vi "FRF_Query.vi"(0 "System no.":i32=1 min=1 max=4 step=1, 2 "Axes to query":string[](array[string]), 3 "All axes?":bool, 4 "Axis identifier?":bool=TRUE, 5 "error in":errorcluster) -> (14 "Referenced?":bool[](array[boolean]), 19 "error out":errorcluster)   [LabVIEW 2020]
doc: "GCS 3.0\n=====\n\nFRF? (Get Referencing Result) \n\nDescription \nQueries whether the axes are referenced.\n\nFormat\nFRF?[ <AxisID>]\n\nArguments\nFRF without arguments starts a reference move for all axes of the controller. The axes start \nsimultaneously.\n<AxisID>\nAn axis of the controller\nThe response to USG? CMD FRF? indicates in the #Related Units block for which axes the \ncommand can be used.\nPossible values: Alias of the axis (p. 94) \n\nResponse\n{<AxisID>\"=\"<Ref_State> LF}\n<Ref_State>\nValue that indicates whether the axis is referenced.\nPossible values:\n0 = Axis is not referenced\n1 = Axis is referenced\n\nExample\n>>frf?\n<<AXIS_1=1\n<<AXIS_2=0\n\nNotes\nWhether the axis is referenced is also displayed in the status register of the axis, which can be \nqueried with the STV? command. \n\nUser command level\nUSR\n\n\nGCS 2.0\n=====\n\nIndicates whether queried axes have been referenced (using REF, FNL, FPL, FRF, MPL, MNL, or - if reference mode is OFF - using POS) successfully or not.\n\nC-413, C-843, C-843.PM, C-866, C-867, C-877, C-880, C-884, C-885, C-886, C-891, E-754, E-861, E-871, E-873, E-874, Hydra, Pollux, Mercury_GCS: If All axes? = TRUE, then Axis identifier? can be FALSE\n\nC-880K005: VI only supported when called through PI_Multix.vi\n\nE-712: If All axes? = TRUE, then Axis identifier? can be FALSE. \n\nE-755: If All axes? = TRUE, then Axis identifier? can be FALSE. Command not available for E-755.101\n\nC-887, F-206, M-8X0: If All axes? = TRUE, then Axis identifier? can be FALSE. Only for GCS syntax version = GCS 2.0 or higher (check with CSV?.vi. If CSV?.vi is not supported, syntax version is GCS 1.0)."
panel:
  # "FRF? (Get Referencing Result)\n\nQueries whether the axes are referenced."
  # "Query"
  # "If all axes: use"
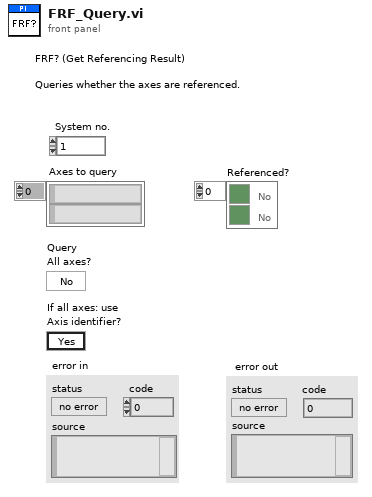
[diagram p1: front panel]
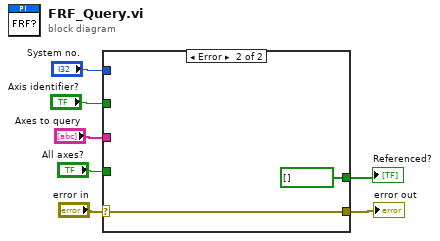
[diagram p0: block diagram]
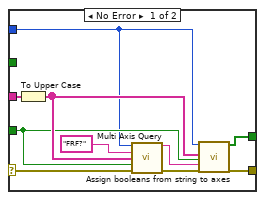
[diagram p2: hidden frame]
diagram:
  n1 = case shown="Error" "error in" {
    selector: "error in" -> [w16 w19]
    tunnel: [w11 bool[] [] ("Booleans")] -> w1
    tunnel: "Axes to query" -> [w17 _]
    tunnel: [w13 w19] -> w2
    tunnel: "System no." -> [w8 _]
    tunnel: "All axes?" -> [w9 _]
    tunnel: "Axis identifier?" -> [_ _]
    frame No Error {
      n2 = To Upper Case(1:w17) -> (0:w12:string[])
      n3 = call "Multi Axis Query.vi"("System no."=w8, "Command"="FRF?", "Axis"=w12, "All axes?"=w9, "error in (no error)"=w16) -> ("Answer"=w10:string, "error out"=w14:errorcluster)  [unwired: 9 in]
      n4 = call "Assign booleans from string to axes.vi"("System no."=w8, "Queried axes"=w12, "All axes queried?"=w9, "Input String"=w10, "error in"=w14) -> ("Booleans"=w11:bool[], "error out"=w13:errorcluster)  [unwired: 13 in]
    }
    frame Error {
      (unwired) string[] [] ("Axes to query out")
    }
  }
  "error out" <- w2
  "Referenced?" <- w1
